vi "Test Double Float.vi"(7 "Name":string="Test Double Float", 8 "Upper Limit":dbl, 9 "Lower Limit":dbl, 10 "Limit Test Type":T1, 11 "Abs_Double Float.lvclass":refnum<class "Abs_Double Float.lvclass">) -> (3 "abs_Node":refnum<class "abs_Node.lvclass">)   [LabVIEW 2021, in "BT.lvlib"]
uses:
  BT.lvlib
  abs_Node/abs_Node.lvclass
  Support/Limit Test Type.ctl
  GitHub/LV_Abstract/Source/Abs_Types/Double Float/Abs_Double Float.lvclass
  C:/Users/Tim/Documents/GitHub/LV_Abstract/Source/Abs_Types/Type/Abs_Type.lvclass
  Test Double Float/Test Double Float.lvclass
  C:/Users/Tim/Documents/LabVIEW/2021/Behaviour Tree/Source/abs_Node/abs_Node.lvclass
  C:/Users/Tim/Documents/LabVIEW/2021/Behaviour Tree/Source/abs_Type Leaf/abs_Type Leaf.lvclass
  abs_Node/abs_Node.lvclass/abs_Node.ctl
  abs_Type Leaf/abs_Type Leaf.lvclass/abs_Type Leaf.ctl
  Test Double Float/Test Double Float.lvclass/Test Double Float.ctl
  abs_Node/Properties/Write Name.vi
  abs_Type Leaf/Properties/Write Value Class.vi
  Test Double Float/Properties/Write Limit Test Type.vi
  Test Double Float/Properties/Write Lower Limit.vi
  Test Double Float/Properties/Write Upper Limit.vi
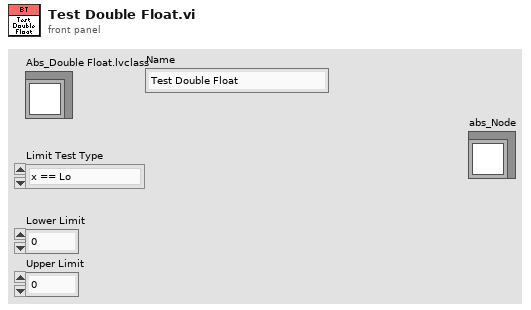
[diagram p1: front panel]
types:
  T1 = typedef "BT.lvlib/Limit Test Type.ctl" = enum16{"x == Lo", "x != Lo", "x > Lo", "x < Lo", "x >= Lo", "x <= Lo", "Lo > x < Hi", "Lo >= x <= Hi", "Lo >= x < Hi", "Lo > x <= Hi", "Lo < x > Hi", "Lo <= x >= Hi", "Lo <= x > Hi", "Lo < x >= Hi", "x == Lo +/- Hi"}
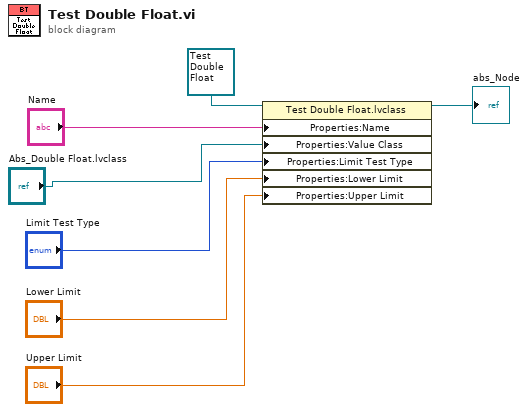
[diagram p0: block diagram]
diagram:
  n1 = property class="Test Double Float.lvclass"(reference=refnum<class "Test Double Float.lvclass"> refnum ("BT.lvlib:Test Double Float.lvclass"), "Properties:Name"="Name", "Properties:Value Class"="Abs_Double Float.lvclass", "Properties:Limit Test Type"="Limit Test Type", "Properties:Lower Limit"="Lower Limit", "Properties:Upper Limit"="Upper Limit") -> (reference out=→"abs_Node":refnum<class "Test Double Float.lvclass">)  [unwired: 1 in, 1 out]
